vi "Trigger.vi"() -> ()   [LabVIEW 2012]
panel:
  in  "Trigger Hysteresis Levels":T1={"Boost A Threshold"=0.0, "Boost A Hyst"=-250.0, "Boost B Threshold"=50.0, "Boost B Hyst"=-150.0, "O2 Threshold"=250.0, "O2 Hyst"=400.0, "Vent Threshold"=50.0, "Vent Hyst"=200.0, "Recirc Threshold "=50.0, "Recirc  Hyst "=-150.0}
  out "Alt States":T2={"Main"=TRUE, "Boost A"=FALSE, "Boost B"=FALSE, "Recirc"=FALSE, "Scrubber"=FALSE, "O2 Valve"=FALSE, "Vent"=FALSE, "Alarm"=FALSE}
  in  "Alt Dif":dbl(slide) scale=-1000.0..1000.0
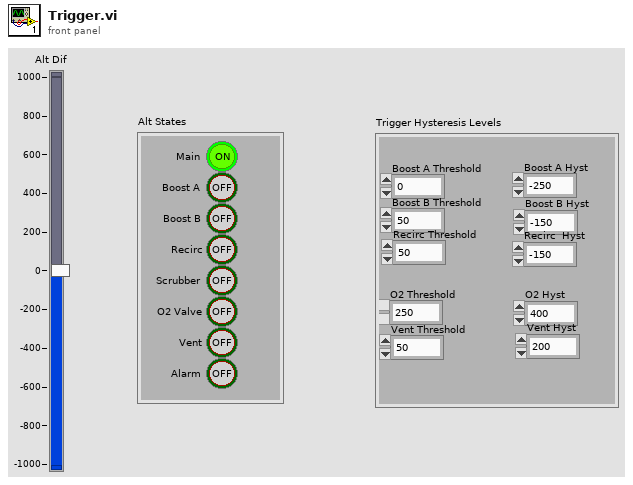
[diagram p1: front panel]
types:
  T1 = cluster{"Boost A Threshold":dbl, "Boost A Hyst":dbl, "Boost B Threshold":dbl, "Boost B Hyst":dbl, "O2 Threshold":dbl, "O2 Hyst":dbl, "Vent Threshold":dbl, "Vent Hyst":dbl, "Recirc Threshold ":dbl, "Recirc  Hyst ":dbl}
  T2 = cluster{"Main":bool, "Boost A":bool, "Boost B":bool, "Recirc":bool, "Scrubber":bool, "O2 Valve":bool, "Vent":bool, "Alarm":bool}
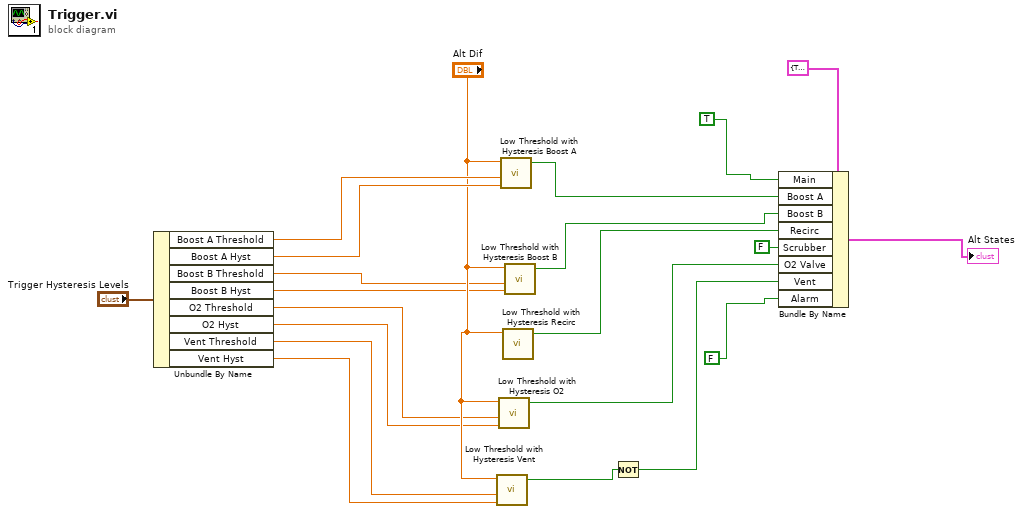
[diagram p0: block diagram]
diagram:
  n1 = Unbundle By Name("Trigger Hysteresis Levels") -> ("Boost A Threshold"=w17:dbl, "Boost A Hyst"=w16:dbl, "Boost B Threshold"=w6:dbl, "Boost B Hyst"=w5:dbl, "O2 Threshold"=w4:dbl, "O2 Hyst"=w3:dbl, "Vent Threshold"=w2:dbl, "Vent Hyst"=w1:dbl)
  n2 = call "Low Threshold with Hysteresis Vent.vi"("Alt Dif"="Alt Dif", "Threshold"=w2, "Hysteresis"=w1) -> ("Boolean"=w8:bool)  [unwired: 3 in, 1 out]
  n3 = call "Low Threshold with Hysteresis O2.vi"("Alt Dif"="Alt Dif", "Threshold"=w4, "Hysteresis"=w3) -> ("Boolean"=w9:bool)  [unwired: 3 in, 1 out]
  n4 = call "Low Threshold with Hysteresis Boost A.vi"("Alt Dif"="Alt Dif", "Threshold"=w17, "Hysteresis"=w16) -> ("Boolean"=w15:bool)  [unwired: 3 in, 1 out]
  n5 = call "Low Threshold with Hysteresis Recirc.vi"("Alt Dif"="Alt Dif") -> ("Boolean"=w12:bool)  [unwired: 5 in, 1 out]
  n6 = call "Low Threshold with Hysteresis Boost B.vi"("Alt Dif"="Alt Dif", "Threshold"=w6, "Hysteresis"=w5) -> ("Boolean"=w13:bool)  [unwired: 4 in]
  n7 = Not(x=w8) -> (.not. x?=w7:bool)
  n8 = Bundle By Name(cluster=T2 {"Main"=TRUE, "Boost A"=FALSE, "Boost B"=FALSE, "Recirc"=FALSE, "Scrubber"=FALSE, "O2 Valve"=FALSE, "Vent"=FALSE, "Alarm"=FALSE} ("Alt States"), "Main"=TRUE, "Boost A"=w15, "Boost B"=w13, "Recirc"=w12, "Scrubber"=FALSE, "O2 Valve"=w9, "Vent"=w7, "Alarm"=FALSE) -> (→"Alt States":T2)
